vi "Set Default Impedance.vi"(8 "error in (no error)":errorcluster, 10 "Default Impedance (0: 50 ohms)":u32(ring) items=["50 ohms", "75 ohms", "90 ohms", "100 ohms", "135 ohms", "150 ohms", "300 ohms", "600 ohms", "900 ohms", "1000 ohms", "1200 ohms"], 11 "VISA resource name":refnum<visa-resource-name>) -> (0 "error out":errorcluster, 3 "VISA resource name out":refnum<visa-resource-name>)   [LabVIEW 2014, in "Fluke 5XXX Series Multicalibrators.lvlib"]
doc: "This VI sets the power-up and reset default impedance used for dBm outputs (ac volts).\n\nNote:\n\nThis VI is available only for instrument model 5520A."
uses:
  Fluke 5XXX Series Multicalibrators.lvlib
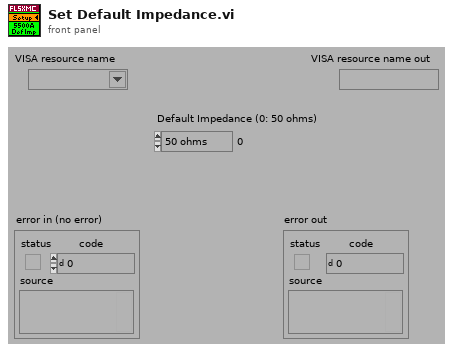
[diagram p1: front panel]
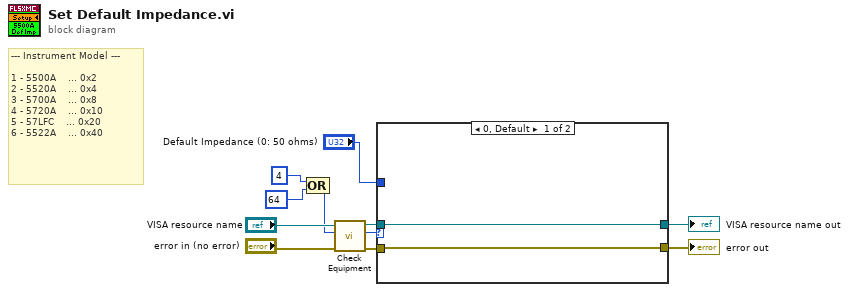
[diagram p0: block diagram]
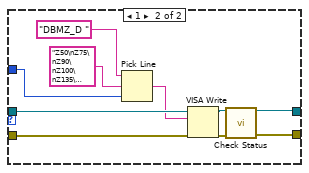
[diagram p2: hidden frame]
diagram:
  # "--- Instrument Model ---\n\n1 - 5500A    ... 0x2\n2 - 5520A    ... 0x4\n3 - 5700A    ... 0x8\n4 - 5720A    ... 0x10\n5 - 57LFC    ... 0x20\n6 - 5522A    ... 0x40"
  n1 = Compound Arithmetic op=OR(4 ("Numeric"), 64 ("Numeric")) -> (w1:i32)
  n2 = call "Check Equipment.vi"("error in (no error)"="error in (no error)", "Bit Mask"=w1, "VISA resource name"="VISA resource name") -> ("error out"=w11:errorcluster, "Present?"=w10:u32, "VISA resource name out"=w9:refnum<visa-resource-name>)  [unwired: 6 in]
  n3 = case shown="0, Default" w10 {
    tunnel: "Default Impedance (0: 50 ohms)" -> [_ w18]
    tunnel: [w12 w14] -> w5
    tunnel: w11 -> [w13 w21]
    tunnel: w9 -> [w12 w20]
    tunnel: [w13 w17] -> w6
    frame 0, Default {
    }
    frame 1 {
      n4 = Pick Line(string ("")="DBMZ_D " ("Reset Command"), multi-line string="Z50\nZ75\nZ90\nZ100\nZ135\nZ150\nZ300\nZ600\nZ900\nZ1000\nZ1200", line index=w18) -> (output string=w19:string)
      n5 = VISA Write(VISA resource name=w20, write buffer=w19, error in (no error)=w21) -> (VISA resource name out=w15:refnum<visa-resource-name>, error out=w16:errorcluster)  [unwired: 1 out]
      n6 = call "Check Status.vi"("VISA resource name"=w15, "error in (no error)"=w16) -> ("VISA resource name out"=w14:refnum<visa-resource-name>, "error out"=w17:errorcluster)  [unwired: 12 in]
    }
  }
  "VISA resource name out" <- w5
  "error out" <- w6
